vi "Steering Control.vi"() -> ()   [LabVIEW 2018]
uses:
  <vilib>/Simulation/Scripting/Companion Diagram/SimConfigNode/SimParams.ctl
  <vilib>/Simulation/Scripting/Companion Diagram/SimConfigNode/_simSolvers.ctl
  <vilib>/Simulation/Implementation/Shared/SIMSCR Execution Mode.ctl
  <vilib>/Platform/TimedLoop/XDataNode/timing_clust.ctl
  <vilib>/Platform/TimedLoop/XDataNode/nitl_modes.ctl
  <vilib>/Platform/TimedLoop/XDataNode/wakeup.ctl
  <vilib>/Simulation/Param Hierarchy/Typedefs/SIMPH Param Control Actions.ctl
  <vilib>/Quanser/Rapid Control Prototyping Toolkit/communications/basic/Basic Stream Receive Mode.ctl
  <vilib>/Quanser/Rapid Control Prototyping Toolkit/communications/basic/Basic Stream Send Mode.ctl
  <vilib>/Simulation/Implementation/Shared/NILVSim_FinalizeModel.vi
  <vilib>/Simulation/Implementation/Shared/NILVSim_FinishedLate.vi
  <vilib>/Simulation/Utility/Implementation/SIM Halt.vi
  <vilib>/Simulation/SignalArithmetic/Implementation/NILVSim Gain.llb/SIM Gain (scalar).vi
  <vilib>/Simulation/Implementation/Shared/NILVSim_Manager.vi
  <vilib>/Simulation/Implementation/Shared/NILVSIM_BeginStep.vi
  <vilib>/Simulation/Implementation/Shared/NILVSim_ParamChanged.vi
  <vilib>/Utility/error.llb/Clear Errors.vi
  <vilib>/Simulation/Implementation/Shared/SIM Unbundle Sim Info.vi
  <vilib>/Simulation/Implementation/Shared/SIMSH Read Queue.vi
  <vilib>/Simulation/Implementation/Shared/NILVSim_Initialize.vi
  <vilib>/Simulation/Utility/Implementation/NILVSim Get Time and IsAcceptedStep.vi
  <vilib>/Simulation/Implementation/Shared/NILVSim_GetModelError.vi
  <vilib>/Simulation/Implementation/Shared/SIM Bundle Sim Info.vi
  <vilib>/Simulation/Scripting/Companion Diagram/SimConfigNode/SimDog.xnode
  SubVIs/Animate.vi
  SubVIs/Auto_Driver.vi
  SubVIs/Track_Model.vi
  SubVIs/Navigation_Sensors_G.vi
  <vilib>/Quanser/Rapid Control Prototyping Toolkit/communications/basic/_TypeSpecific/CL Comm Basic Stream Client (DBL).vi
  <vilib>/Quanser/Rapid Control Prototyping Toolkit/communications/basic/CL Comm Basic Stream Client.vi
  <vilib>/Quanser/Rapid Control Prototyping Toolkit/visualization/Visualization.lvclass
  <vilib>/Platform/TimedLoop/XDataNode/XDataNode.xnode
  <vilib>/Simulation/Implementation/XNodeFramework/SimXNode/SimX.xnode
  <vilib>/Platform/TimedLoop/XDataNode/XDNodeRunTimeDep.lvlib
  <vilib>/Simulation/Implementation/Shared/NI_SIM_Implementation.lvlib
panel:
  out "Steering Response":cluster{"output":dbl, "Desired_Speed":dbl}(graph)={"output"=0.05835237992894671, "Desired_Speed"=0.06134}
  in  "Steer Kd":dbl=0.1
  in  "Steer Kp":dbl=1.0
  out "Speed (km/h)":dbl(knob)=70.10395687848734 scale=0.0..200.0
  out "Steering Angle (rad)":dbl(knob)=0.06134 scale=2.0..-2.0
  in  "Stop":bool caption="START"
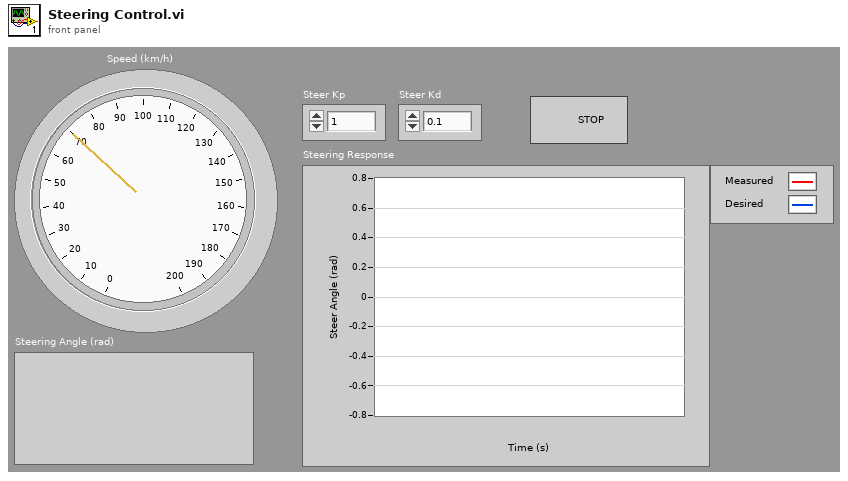
[diagram p1: front panel]
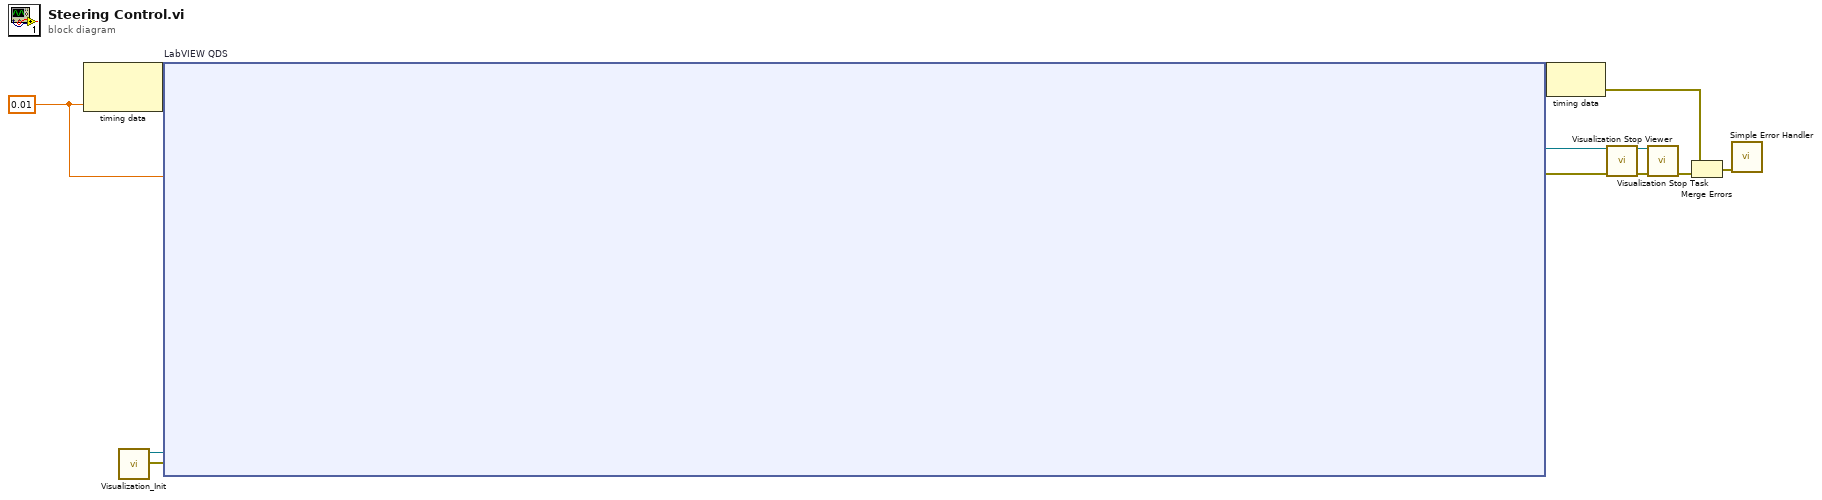
[diagram p0: block diagram]
diagram:
  w1 = 0.01 ("Step Size (s)")
  n1 = node-c288(w1) -> (w12:variant)  [unwired: 1 in]
  n2 = call "Visualization_Init.vi"() -> ("error out"=w9:errorcluster, "visualization out"=w10:refnum<class "Visualization.lvclass">)  [unwired: 10 in]
  n3 = node-c254 "LabVIEW QDS"(w12, w10, w9, w1) -> (w11:variant, w3:errorcluster, w4:refnum<class "Visualization.lvclass">)
  n4 = node-c288(w11) -> (w7:errorcluster)
  n5 = call <vilib>:"Visualization Stop Viewer.vi"("visualization in"=w4, "error in (no error)"=w3) -> ("visualization out"=w6:refnum<class "Visualization.lvclass">, "error out"=w5:errorcluster)  [unwired: 12 in]
  n6 = call <vilib>:"Visualization Stop Task.vi"("visualization in"=w6, "error in (no error)"=w5) -> ("error out"=w2:errorcluster)  [unwired: 13 in]
  n7 = Merge Errors(w7, w2) -> (w8:errorcluster)
  n8 = call <vilib>:"Simple Error Handler.vi"("error in (no error)"=w8) -> ()  [unwired: 4 in, 5 out]
